vi "Get Status Channels.vi"(8 "error in (no error)":errorcluster, 11 "Item Ref in":T1 format="%.0x") -> (0 "error out":errorcluster, 2 "Channels refs":T1[](array[typedef]) format="%.0x", 3 "Item Ref out":T1 format="%.0x")   [LabVIEW 2017, in "DSF Shared.lvlib"]
uses:
  Shared/DSF Shared.lvlib
  <vilib>/NI Veristand/Custom Device API/Custom Device Item Ref.ctl
  <vilib>/NI Veristand/Custom Device API/Custom Device API.lvlib
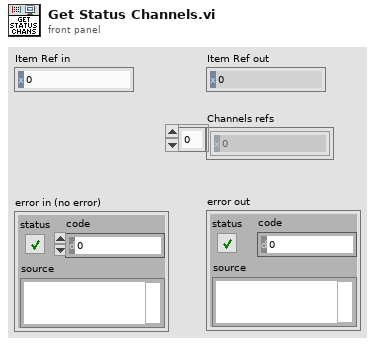
[diagram p1: front panel]
types:
  T1 = typedef "Custom Device API.lvlib/Custom Device Item Ref.ctl" = u64
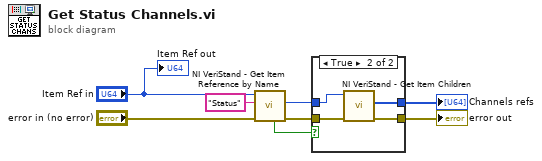
[diagram p0: block diagram]
diagram:
  n1 = call <vilib>:"NI VeriStand - Get Item Reference by Name.vi"("error in (no error)"="error in (no error)", "Item Name"="Status", "Parent Ref in"="Item Ref in") -> ("error out"=w7:errorcluster, "Item Ref"=w5:T1, "Found"=w1:bool)  [unwired: 5 in, 1 out]
  n2 = case shown="True" w1 {
    tunnel: w7 -> [w9 w13]
    tunnel: w5 -> [_ w12]
    tunnel: [w9 w11] -> w4
    tunnel: [_ w10] -> w3
    frame False {
    }
    frame True {
      n3 = call <vilib>:"NI VeriStand - Get Item Children.vi"("error in (no error)"=w13, "Item Ref in"=w12) -> ("error out"=w11:errorcluster, "Child Refs"=w10:T1[])  [unwired: 6 in, 2 out]
    }
  }
  "error out" <- w4
  "Channels refs" <- w3
  "Item Ref out" <- "Item Ref in"
